vi "Autonomous Independent.vi"   [LabVIEW 2017]
doc: "This VI is called when autonomous begins, and will automatically be terminated when autonomous ends. You can carry out timed or sensor driven robot movement independently without needing to return to the caller."
uses:
  <vilib>/Rock Robotics/WPI/Utilities/WPI_GetSetVariantRefNum.vi
  <vilib>/Rock Robotics/Network Tables/NT Write Numeric Array.vi
  <vilib>/Rock Robotics/Network Tables/NT Read Number.vi
  <vilib>/Rock Robotics/WPI/RobotDrive/WPI_RobotDriveArcadeDrive_Standard(NoSaturation).vi
  <vilib>/Rock Robotics/Network Tables/NT Read Boolean.vi
  <vilib>/Rock Robotics/Network Tables/NT Write String.vi
panel:
  # "Be sure to right-click and choose Data Operations>>Make Current Value default if you want to save the array values with the VI"
types:
  T1 = typedef "WPI_GyroDevRef.ctl" = cluster{"DevStatus":errorcluster, "Analog Channel":T2, "Gain (VoltsPerDegree/Second)":dbl, "Gyro Type":enum16{"Analog", "XRS450"}, "Handle":i32, "SPI Bus":T3, "Device Found":bool, "Sample Rate":dbl, "Calibrate On Open":bool, "Offset":dbl}
  T2 = typedef "FPGA_AIChannel.ctl" = enum8{"AI 0", "AI 1", "AI 2", "AI 3", "AI MXP 0", "AI MXP 1", "AI MXP 2", "AI MXP 3", "Invalid"}
  T3 = typedef "spi_bus.ctl" = enum16{"SPI On-Board, CS0", "SPI On-Board, CS1", "SPI On-Board, CS2", "SPI On-Board, CS3", "SPI MXP", "Invalid"}
  T4 = typedef "WPI_JoystickDevRef.ctl" = cluster{"Device":T5}
  T5 = typedef "WPI_JoystickDeviceEnum.ctl" = enum16{"USB 0", "USB 1", "USB 2", "USB 3", "USB 4", "USB 5"}
  T6 = typedef "WPI_RobotDriveDevRef.ctl" = cluster{"DevStatus":errorcluster, "Motors[]":T7[], "Square Inputs":bool, "Max Output":dbl}
  T7 = typedef "WPI_MotorControlDeviceRef.ctl" = cluster{"DeviceStatus":errorcluster, "Type":T8, "PWM":cluster{"PWM Channel":T9, "DeadBand":T10}, "CAN":cluster{"Device Number":u8, "SetOutput VI Ref":variant, "GetOutput VI Ref":variant, "Enable VI Ref":variant, "Disable VI Ref":variant, "Data":variant}, "Invert":bool, "DIO PWM":cluster{"PWM \"Enable\" Channel":T9, "DIOChannel":T11, "PWM Rate":dbl}}
  T8 = typedef "WPI_MotorControlType.ctl" = enum16{"PWM", "CAN", "DIO PWM"}
  T9 = typedef "FPGA_DIOPWMChannel.ctl" = enum8{"PWM 0", "PWM 1", "PWM 2", "PWM 3", "PWM 4", "PWM 5", "PWM 6", "PWM 7", "PWM 8", "PWM 9", "PWM MXP 0", "PWM MXP 1", "PWM MXP 2", "PWM MXP 3", "PWM MXP 4", "PWM MXP 5", "PWM MXP 6", "PWM MXP 7", "PWM MXP 8", "PWM MXP 9", "Invalid"}
  T10 = typedef "WPI_PWMDeadband.ctl" = cluster{"Name":string, "maxPositivePwm":i32, "minPositivePwm":i32, "centerPwm":i32, "maxNegativePwm":i32, "minNegativePwm":i32, "angularRange":u16}
  T11 = typedef "FPGA_DIOChannel.ctl" = enum8{"DIO 0", "DIO 1", "DIO 2", "DIO 3", "DIO 4", "DIO 5", "DIO 6", "DIO 7", "DIO 8", "DIO 9", "DIO MXP 0", "DIO MXP 1", "DIO MXP 2", "DIO MXP 3", "DIO MXP 4", "DIO MXP 5", "DIO MXP 6", "DIO MXP 7", "DIO MXP 8", "DIO MXP 9", "DIO MXP 10", "DIO MXP 11", "DIO MXP 12", "DIO MXP 13", "DIO MXP 14", "DIO MXP 15", "SPI Port CS1", "SPI Port CS2", "SPI Port CS3", "SPI Port MISO", "SPI Port MOSI", "Invalid"}
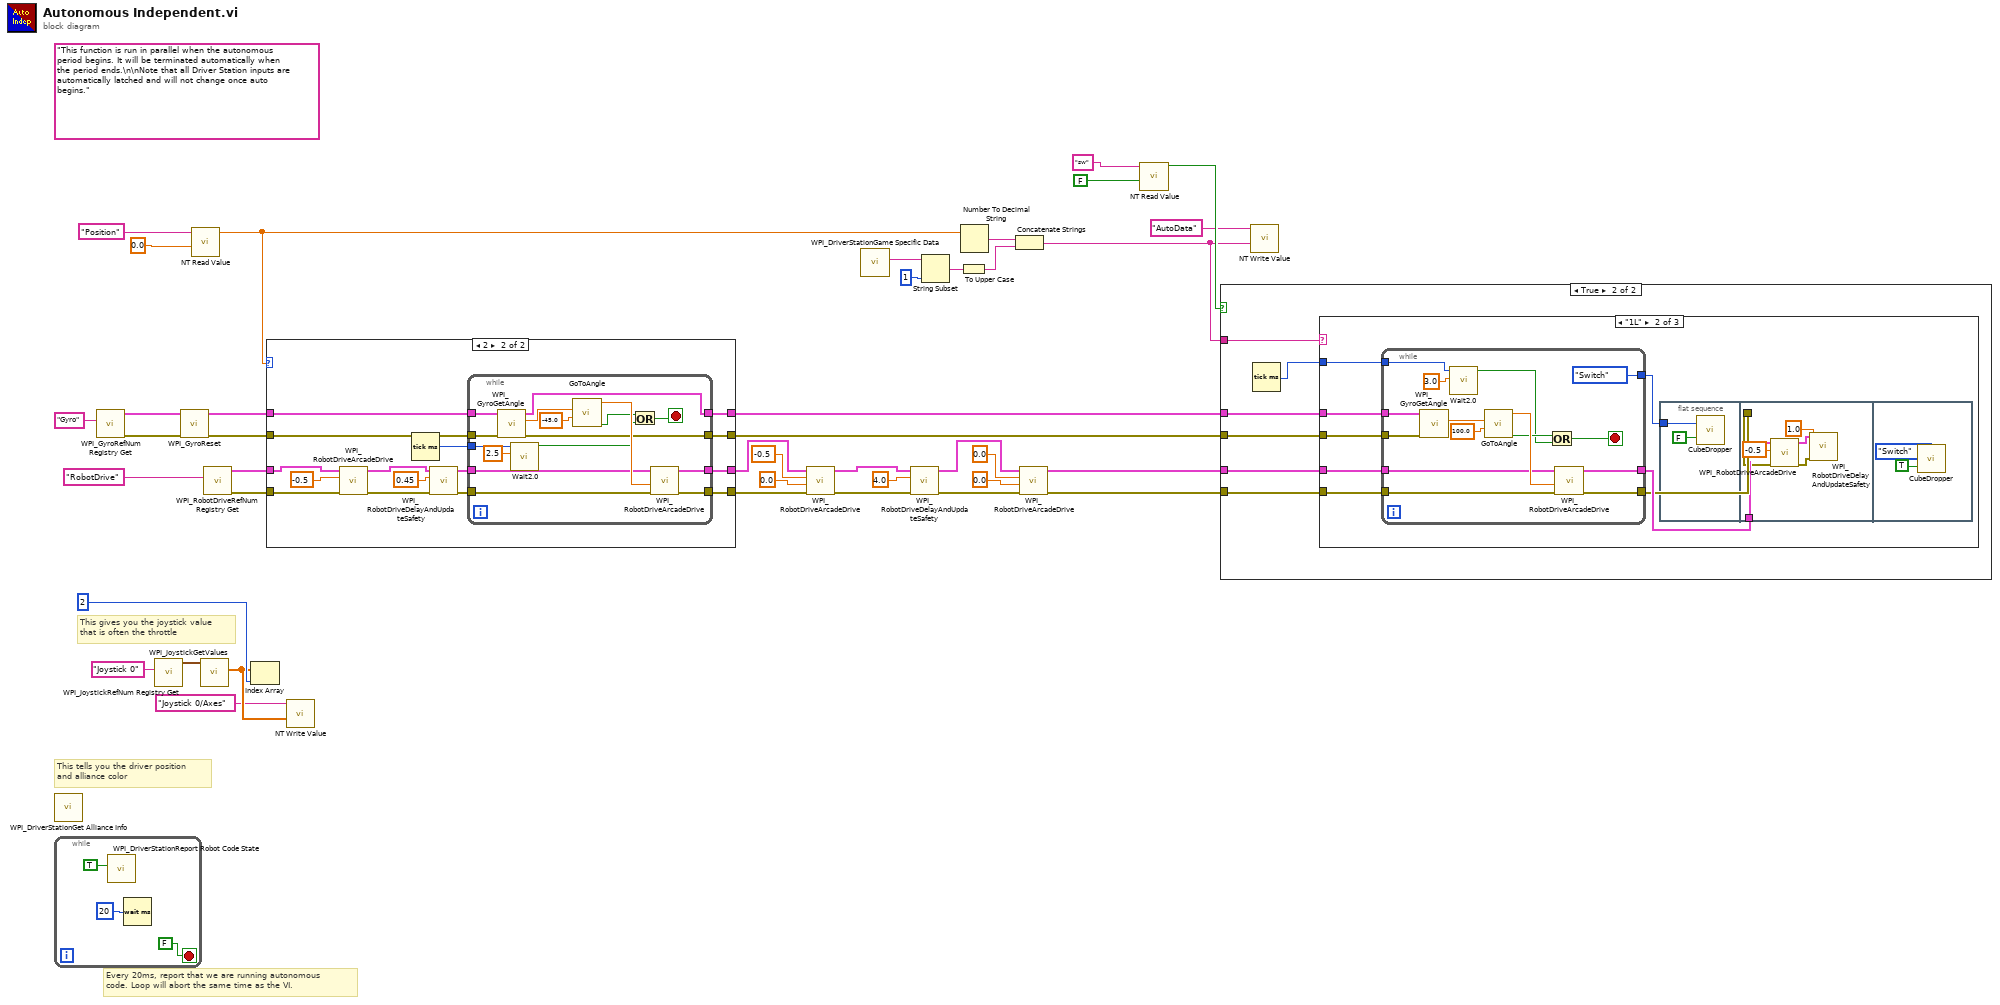
[diagram p0: block diagram]
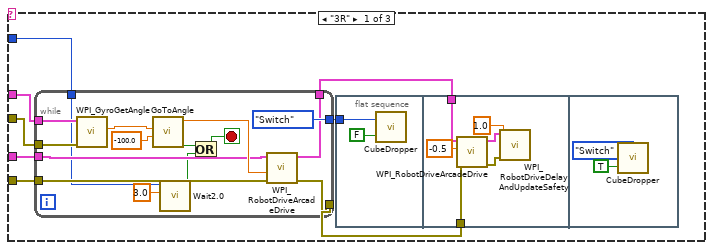
[diagram p3: hidden frame]
diagram:
  (unwired) "This function is run in parallel when the autonomous period begins. It will be terminated automatically when the period ends.\n\nNote that all Driver Station inputs are automatically latched and will not change once auto begins."
  # "Every 20ms, report that we are running autonomous\ncode. Loop will abort the same time as the VI."
  # "This gives you the joystick value\nthat is often the throttle"
  # "This tells you the driver position\nand alliance color"
  n1 = call <vilib>:"WPI_DriverStationGet Alliance Info.vi"() -> ()  [unwired: 12 out]
  n2 = while {
    stop <- FALSE stop-if-true
    n3 = call <vilib>:"WPI_DriverStationReport Robot Code State.vi"("Autonomous"=TRUE) -> ()  [unwired: 10 in, 1 out]
    n4 = Wait (ms)(milliseconds to wait=u32 20) -> ()  [unwired: 1 out]
  }
  n5 = call <vilib>:"WPI_GyroRefNum Registry Get.vi"("refnum name"="Gyro") -> ("error out"=w18:errorcluster, "GyroDevRef"=w21:T1)  [unwired: 9 in]
  n6 = call <vilib>:"WPI_JoystickRefNum Registry Get.vi"("refnum name"="Joystick 0") -> ("JoystickDevRef"=w40:T4)  [unwired: 1 in, 9 out]
  n7 = call <vilib>:"WPI_GyroReset.vi"("error in (no error)"=w18, "GyroDevRef"=w21) -> ("error out"=w19:errorcluster, "GyroDevRef"=w20:T1)  [unwired: 8 in]
  n8 = call-poly <vilib>:"NT Read Value.vi"("Default Value"=0.0, "Name"="Position") -> ("Numeric"=w3:dbl)  [unwired: 8 in, 1 out]
  n9 = call <vilib>:"WPI_JoystickGetValues.vi"("JoystickDevRef"=w40) -> ("Axes"=w38:dbl[])  [unwired: 6 in, 4 out]
  n10 = call <vilib>:"WPI_RobotDriveRefNum Registry Get.vi"("refnum name"="RobotDrive") -> ("error out"=w23:errorcluster, "RobotDriveDevRef"=w26:T6)  [unwired: 9 in]
  n11 = Index Array(array=w38, index=2) -> ()  [unwired: 1 out]
  n12 = case shown="2" w3 {
    tunnel: w26 -> [w48 w59]
    tunnel: [w48 w63] -> w25
    tunnel: [w47 w62] -> w24
    tunnel: w23 -> [w47 w58]
    tunnel: w20 -> [w46 w61]
    tunnel: w19 -> [w45 w60]
    tunnel: [w45 w51] -> w9
    tunnel: [w46 w50] -> w8
    frame 0, Default {
    }
    frame 2 {
      n13 = call-poly <vilib>:"WPI_RobotDriveArcadeDrive.vi"("error in (no error)"=w58, "X axis value"=-0.5, "RobotDriveDevRef"=w59) -> ("error out"=w55:errorcluster, "RobotDriveDevRef"=w56:T6)  [unwired: 6 in, 1 out]
      n14 = Tick Count (ms)() -> (millisecond timer value=w49:u32)
      n15 = call <vilib>:"WPI_RobotDriveDelayAndUpdateSafety.vi"("error in (no error)"=w55, "Delay (s)"=0.45, "RobotDriveDevRef"=w56) -> ("error out"=w52:errorcluster, "RobotDriveDevRef 2"=w53:T6)  [unwired: 7 in]
      n16 = while {
        tunnel: [w76] -> w63
        tunnel: [w75] -> w62
        tunnel: w61 -> [w74]
        tunnel: w60 -> [w73]
        tunnel: w53 -> [w72]
        tunnel: w52 -> [w71]
        tunnel: [w70] -> w51
        tunnel: [w69] -> w50
        tunnel: w49 -> [w68]
        stop <- w66 stop-if-true
        n17 = call <vilib>:"WPI_GyroGetAngle.vi"("error in (no error)"=w73, "GyroDevRef"=w74) -> ("error out"=w70:errorcluster, "Angle"=w77:dbl, "GyroDevRef"=w69:T1)  [unwired: 6 in, 1 out]
        n18 = call "Wait2.0.vi"("Seconds"=2.5, "Start Time"=w68) -> ("Output"=w64:bool)  [unwired: 9 in]
        n19 = call "GoToAngle.vi"("Target Angle"=-45.0, "Angle"=w77) -> ("AtTarget"=w65:bool, "X axis"=w79:dbl)  [unwired: 8 in]
        n20 = Or(x=w65, y=w64) -> (x .or. y?=w66:bool)
        n21 = call-poly <vilib>:"WPI_RobotDriveArcadeDrive.vi"("error in (no error)"=w71, "Y axis value"=w79, "RobotDriveDevRef"=w72) -> ("error out"=w75:errorcluster, "RobotDriveDevRef"=w76:T6)  [unwired: 6 in, 1 out]
      }
    }
  }
  n22 = call-poly <vilib>:"NT Write Value.vi"("Numeric Array"=w38, "Name"="Joystick 0/Axes") -> ()  [unwired: 9 in, 1 out]
  n23 = call-poly <vilib>:"WPI_RobotDriveArcadeDrive.vi"("error in (no error)"=w24, "Y axis value"=0.0, "X axis value"=-0.5, "RobotDriveDevRef"=w25) -> ("error out"=w34:errorcluster, "RobotDriveDevRef"=w35:T6)  [unwired: 5 in, 1 out]
  n24 = call <vilib>:"WPI_DriverStationGame Specific Data.vi"() -> ("Game Specific Data"=w14:string)  [unwired: 11 in]
  n25 = call <vilib>:"WPI_RobotDriveDelayAndUpdateSafety.vi"("error in (no error)"=w34, "Delay (s)"=4.0, "RobotDriveDevRef"=w35) -> ("error out"=w32:errorcluster, "RobotDriveDevRef 2"=w33:T6)  [unwired: 7 in]
  n26 = String Subset(string=w14, length (rest)=1 ("length (rest)")) -> (substring=w11:string)  [unwired: 1 in]
  n27 = To Upper Case(1:w11) -> (0:w12:string)
  n28 = Number To Decimal String(number=w3) -> (decimal integer string=w13:string)  [unwired: 1 in]
  n29 = Concatenate Strings(w13, w12) -> (w1:string)
  n30 = call-poly <vilib>:"WPI_RobotDriveArcadeDrive.vi"("error in (no error)"=w32, "Y axis value"=0.0 ("Right axis value"), "X axis value"=0.0 ("Left axis value"), "RobotDriveDevRef"=w33) -> ("error out"=w7:errorcluster, "RobotDriveDevRef"=w10:T6)  [unwired: 5 in, 1 out]
  n31 = call-poly <vilib>:"NT Read Value.vi"("Default Value"=FALSE, "Name"="sw") -> ("Boolean"=w4:bool)  [unwired: 8 in, 1 out]
  n32 = case shown="True" w4 {
    tunnel: w1 -> [_ w85]
    tunnel: w10 -> [_ w84]
    tunnel: w9 -> [_ w83]
    tunnel: w8 -> [_ w82]
    tunnel: w7 -> [_ w81]
    frame False {
    }
    frame True {
      n33 = Tick Count (ms)() -> (millisecond timer value=w80:u32)
      n34 = case shown="\"1L\"" w85 {
        tunnel: w84 -> [w93 w126 _]
        tunnel: w83 -> [w92 w125 _]
        tunnel: w82 -> [w91 w124 _]
        tunnel: w81 -> [w90 w123 _]
        tunnel: w80 -> [w88 w122 _]
        frame "3R" {
          n35 = while {
            tunnel: w91 -> [w115]
            tunnel: w92 -> [w114]
            tunnel: w93 -> [w113]
            tunnel: w90 -> [w112]
            tunnel: [enum16{"Switch", "Scale", "Bottom", "Null"}."Switch" ("Height")] -> w89
            tunnel: w88 -> [w107]
            tunnel: [w105] -> w87
            tunnel: [w104] -> w86
            stop <- w110 stop-if-true
            n36 = call <vilib>:"WPI_GyroGetAngle.vi"("error in (no error)"=w114, "GyroDevRef"=w115) -> ("Angle"=w116:dbl)  [unwired: 6 in, 3 out]
            n37 = call "GoToAngle.vi"("Target Angle"=-100.0, "Angle"=w116) -> ("AtTarget"=w109:bool, "X axis"=w118:dbl)  [unwired: 8 in]
            n38 = call "Wait2.0.vi"("Seconds"=3.0, "Start Time"=w107) -> ("Output"=w108:bool)  [unwired: 9 in]
            n39 = Or(x=w109, y=w108) -> (x .or. y?=w110:bool)
            n40 = call-poly <vilib>:"WPI_RobotDriveArcadeDrive.vi"("error in (no error)"=w112, "Y axis value"=w118, "RobotDriveDevRef"=w113) -> ("error out"=w105:errorcluster, "RobotDriveDevRef"=w104:T6)  [unwired: 6 in, 1 out]
          }
          n41 = flat-sequence {
            tunnel: w89 -> [w95]
            tunnel: w87 -> [w101]
            tunnel: w86 -> [w100]
            frame #0 {
              n42 = call "CubeDropper.vi"("Shoot"=FALSE, "Height"=w95) -> ()  [unwired: 1 out]
            }
            frame #1 {
              n43 = call-poly <vilib>:"WPI_RobotDriveArcadeDrive.vi"("error in (no error)"=w101, "X axis value"=-0.5, "RobotDriveDevRef"=w100) -> ("error out"=w97:errorcluster, "RobotDriveDevRef"=w98:T6)  [unwired: 6 in, 1 out]
              n44 = call <vilib>:"WPI_RobotDriveDelayAndUpdateSafety.vi"("error in (no error)"=w97, "Delay (s)"=1.0, "RobotDriveDevRef"=w98) -> ()  [unwired: 7 in, 2 out]
            }
            frame #2 {
              n45 = call "CubeDropper.vi"("Shoot"=TRUE, "Height"=enum16{"Switch", "Scale", "Bottom", "Null"}."Switch") -> ()  [unwired: 1 out]
            }
          }
        }
        frame "1L" {
          n46 = while {
            tunnel: [w148] -> w120
            tunnel: [w147] -> w119
            tunnel: w124 -> [w146]
            tunnel: w125 -> [w145]
            tunnel: w126 -> [w144]
            tunnel: w123 -> [w143]
            tunnel: [enum16{"Switch", "Scale", "Bottom", "Null"}."Switch" ("Height")] -> w121
            tunnel: w122 -> [w137]
            stop <- w140 stop-if-true
            n47 = call <vilib>:"WPI_GyroGetAngle.vi"("error in (no error)"=w145, "GyroDevRef"=w146) -> ("Angle"=w149:dbl)  [unwired: 6 in, 3 out]
            n48 = call "Wait2.0.vi"("Seconds"=3.0, "Start Time"=w137) -> ("Output"=w138:bool)  [unwired: 9 in]
            n49 = call "GoToAngle.vi"("Target Angle"=100.0, "Angle"=w149) -> ("AtTarget"=w139:bool, "X axis"=w151:dbl)  [unwired: 8 in]
            n50 = Or(x=w139, y=w138) -> (x .or. y?=w140:bool)
            n51 = call-poly <vilib>:"WPI_RobotDriveArcadeDrive.vi"("error in (no error)"=w143, "Y axis value"=w151, "RobotDriveDevRef"=w144) -> ("error out"=w147:errorcluster, "RobotDriveDevRef"=w148:T6)  [unwired: 6 in, 1 out]
          }
          n52 = flat-sequence {
            tunnel: w121 -> [w127]
            tunnel: w120 -> [w130]
            tunnel: w119 -> [w129]
            frame #0 {
              n53 = call "CubeDropper.vi"("Shoot"=FALSE, "Height"=w127) -> ()  [unwired: 1 out]
            }
            frame #1 {
              n54 = call-poly <vilib>:"WPI_RobotDriveArcadeDrive.vi"("error in (no error)"=w129, "X axis value"=-0.5, "RobotDriveDevRef"=w130) -> ("error out"=w132:errorcluster, "RobotDriveDevRef"=w133:T6)  [unwired: 6 in, 1 out]
              n55 = call <vilib>:"WPI_RobotDriveDelayAndUpdateSafety.vi"("error in (no error)"=w132, "Delay (s)"=1.0, "RobotDriveDevRef"=w133) -> ()  [unwired: 7 in, 2 out]
            }
            frame #2 {
              n56 = call "CubeDropper.vi"("Shoot"=TRUE, "Height"=enum16{"Switch", "Scale", "Bottom", "Null"}."Switch") -> ()  [unwired: 1 out]
            }
          }
        }
        frame Default {
        }
      }
    }
  }
  n57 = call-poly <vilib>:"NT Write Value.vi"("String"=w1, "Name"="AutoData") -> ()  [unwired: 9 in, 1 out]
